vi "telemetry_beta.vi"() -> ()   [LabVIEW 2017]
uses:
  <vilib>/nican/nican.llb/ncNetAttr.ctl
  <vilib>/Platform/TimedLoop/XDataNode/XDataNode.xnode
  <vilib>/Platform/TimedLoop/XDataNode/nitl_modes.ctl
  <vilib>/Platform/TimedLoop/XDataNode/XDNodeRunTimeDep.lvlib
  <vilib>/Platform/TimedLoop/XDataNode/wakeup.ctl
  <vilib>/Platform/TimedLoop/XDataNode/timing_clust.ctl
panel:
  out "output cluster":T1
  in  "CAN1 Enable":bool
  in  "STOP":bool
  out "Error CAN1":errorcluster {"code" format="%.0x"}
  out "Error CAN0":errorcluster {"code" format="%.0x"}
  in  "Communication":u16(ring) items=["WiFi", "NI CAN", "NI XCAN"]
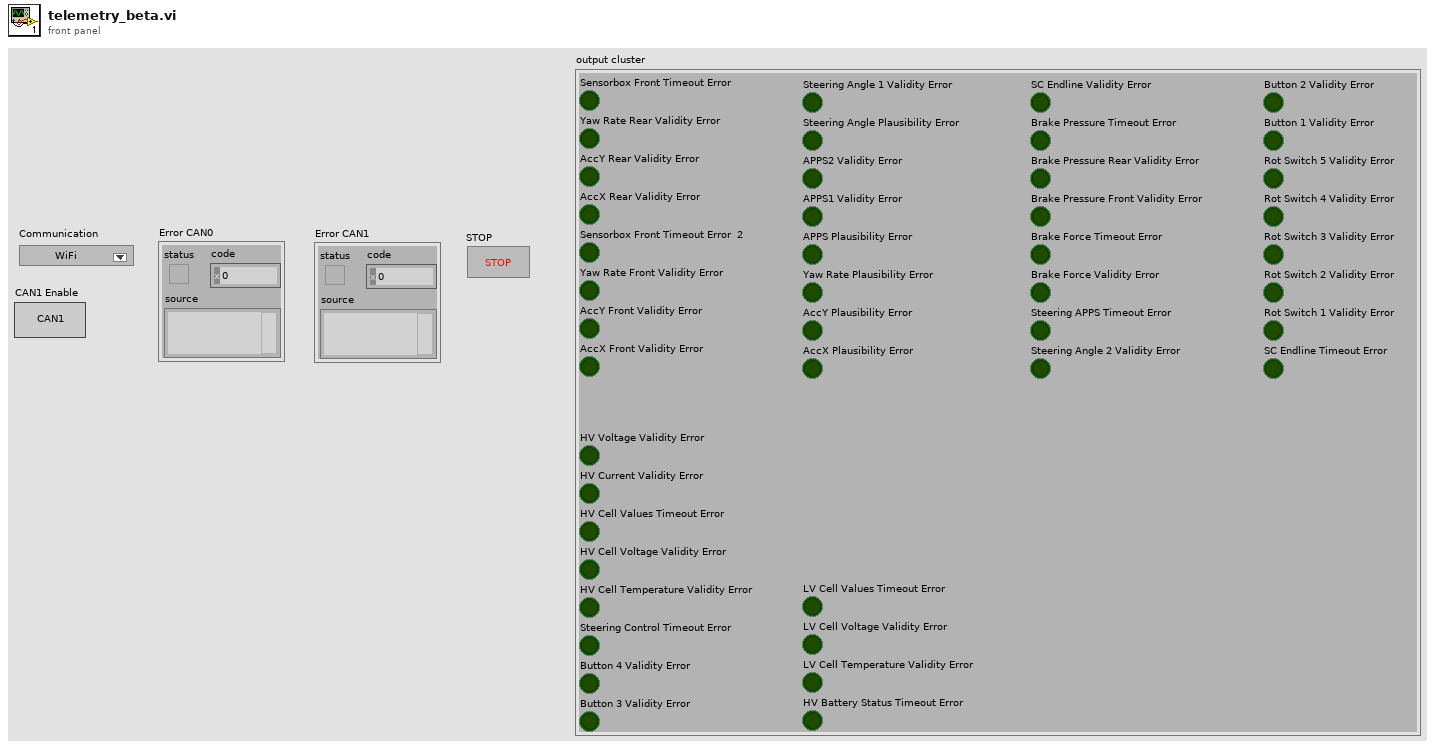
[diagram p1: front panel]
types:
  T1 = cluster{"Sensorbox Front Timeout Error ":bool, "Yaw Rate Rear Validity Error ":bool, "AccY Rear Validity Error":bool, "AccX Rear Validity Error ":bool, "Sensorbox Front Timeout Error  2":bool, "Yaw Rate Front Validity Error":bool, "AccY Front Validity Error":bool, "AccX Front Validity Error":bool, "Steering Angle 1 Validity Error":bool, "Steering Angle Plausibility Error":bool, "APPS2 Validity Error":bool, "APPS1 Validity Error":bool, "APPS Plausibility Error ":bool, "Yaw Rate Plausibility Error ":bool, "AccY Plausibility Error ":bool, "AccX Plausibility Error ":bool, "SC Endline Validity Error":bool, "Brake Pressure Timeout Error ":bool, "Brake Pressure Rear Validity Error":bool, "Brake Pressure Front Validity Error":bool, "Brake Force Timeout Error ":bool, "Brake Force Validity Error ":bool, "Steering APPS Timeout Error":bool, "Steering Angle 2 Validity Error":bool, "Button 2 Validity Error":bool, "Button 1 Validity Error":bool, "Rot Switch 5 Validity Error":bool, "Rot Switch 4 Validity Error":bool, "Rot Switch 3 Validity Error":bool, "Rot Switch 2 Validity Error":bool, "Rot Switch 1 Validity Error":bool, "SC Endline Timeout Error":bool, "HV Voltage Validity Error":bool, "HV Current Validity Error":bool, "HV Cell Values Timeout Error":bool, "HV Cell Voltage Validity Error":bool, "HV Cell Temperature Validity Error":bool, "Steering Control Timeout Error":bool, "Button 4 Validity Error":bool, "Button 3 Validity Error":bool, "LV Cell Values Timeout Error":bool, "LV Cell Voltage Validity Error":bool, "LV Cell Temperature Validity Error":bool, "HV Battery Status Timeout Error":bool}
  T2 = typedef "ncNetAttr.ctl" = cluster{"Start On Open":enum32{"FALSE", "TRUE"}, "Baud Rate":u32, "Read Queue Length":u32, "Write Queue Length":u32, "Standard Comparator":u32, "Standard Mask":u32, "Extended Comparator":u32, "Extended Mask":u32}
  T3 = typedef "xobjhandle.ctl" = u32
  T4 = cluster{"ObjHandle CAN0":T3, "Error CAN0":errorcluster, "Error CAN1":errorcluster, "ObjHandle CAN1":T3, "Double":bool}
  T5 = typedef "XDNodeRunTimeDep.lvlib/timing_clust.ctl" = cluster{"Expected End [f-1]":u64, "Actual End [f-1]":u64, "Finished Late? [f-1]":bool, "Expected End [i-1]":u64, "Actual End [i-1]":u64, "Finished Late? [i-1]":bool, "Expected Start [i]":u64, "Actual Start [i]":u64, "Expected Start [f]":u64, "Actual Start [f]":u64, "Source Name":string, "Structure Name":string, "Period":i64, "Deadline":i64, "Offset":i64, "Start":i64, "Priority":i32, "Timeout":i32, "Mode":T6, "Wakeup Reason":T7, "Error":errorcluster, "Source Type":string, "Secondary Source Type":string, "Global End Time":u64, "Global Start Time":u64, "Frame Duration":u64, "Iteration Duration":u64, "Assigned CPU":i32, "I/O Scan Engine Mode":u32}
  T6 = typedef "XDNodeRunTimeDep.lvlib/nitl_modes.ctl" = enum32{"No Change", "Process missed periods, maintain original phase", "Discard missed periods, maintain original phase", "Process missed periods, ignore original phase", "Discard missed periods, ignore original phase"}
  T7 = typedef "XDNodeRunTimeDep.lvlib/wakeup.ctl" = enum32{"Normal", "Aborted", "Asynchronous wakeup", "Timing source error", "Timed loop error", "Timeout"}
  T8 = typedef "CanFrameTimed.ctl" = cluster{"Timestamp":dbl, "ArbitrationId":u32, "IsRemote":u8, "DataLength":u8, "Data":u8[]}
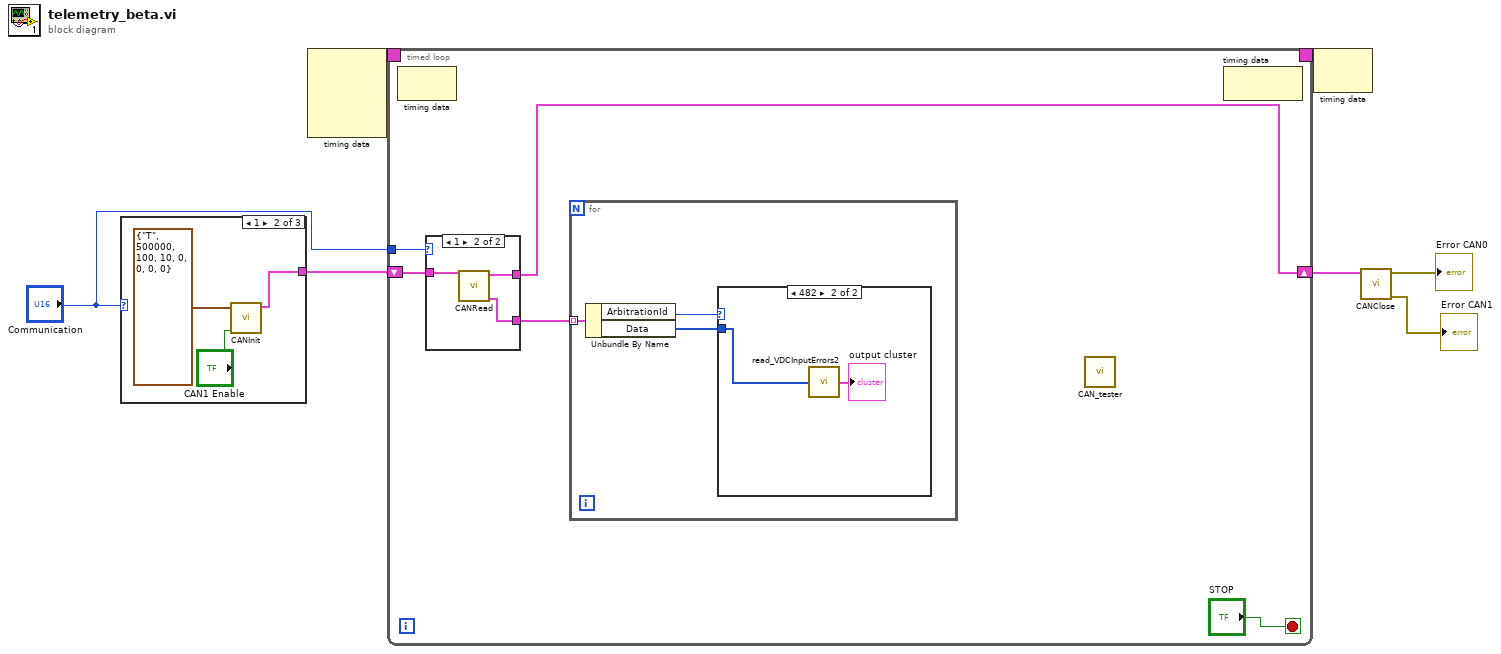
[diagram p0: block diagram]
diagram:
  n1 = case shown="1" "Communication" {
    tunnel: [_ w9 _] -> w5
    frame 0, Default {
    }
    frame 1 {
      n2 = call "CANInit.vi"("CAN1 Enable"="CAN1 Enable", "CAN Network Interface Config"=T2 {"Start On Open"=enum."TRUE", "Baud Rate"=500000, "Read Queue Length"=100, "Write Queue Length"=10, "Standard Comparator"=0, "Standard Mask"=0, "Extended Comparator"=0, "Extended Mask"=0}) -> ("Double CAN"=w9:T4)  [unwired: 9 in]
    }
    frame 2 {
    }
  }
  n3 = node-c288() -> (w7:T5)  [unwired: 4 in]
  n4 = timed-loop {
    timing: w7 -> [_]
    timing-out: [_] -> w6
    shift-right: [w14] -> w3
    shift-left: w5 -> [w15]
    tunnel: "Communication" -> [w13]
    stop <- "STOP" stop-if-true
    n5 = node-c288() -> ()  [unwired: 1 in, 1 out]
    n6 = case shown="1" w13 {
      tunnel: w15 -> [w21 w24]
      tunnel: [w21 w23] -> w14
      tunnel: [_ w22] -> w11
      frame 0, Default {
      }
      frame 1 {
        n7 = call "CANRead.vi"("Double CAN in"=w24) -> ("Data"=w22:T8[], "Double CAN out"=w23:T4)  [unwired: 9 in]
      }
    }
    n8 = for {
      tunnel: w11 -> [w18] mode=indexing
      n9 = Unbundle By Name(w18) -> ("ArbitrationId"=w17:u32, "Data"=w16:u8[])
      n10 = case shown="482" w17 {
        tunnel: w16 -> [_ w20]
        frame 0, Default {
        }
        frame 1154 {
          n11 = call "read_VDCInputErrors2.vi"("Array"=w20) -> ("output cluster"=→"output cluster":T1)
        }
      }
    }
    n12 = call "CAN_tester.vi"() -> ()  [unwired: 12 in]
    n13 = node-c288() -> ()  [unwired: 1 in, 1 out]
  }
  n14 = node-c288(w6) -> ()  [unwired: 1 out]
  n15 = call "CANClose.vi"("Double CAN in"=w3) -> ("Error CAN1"=→"Error CAN1":errorcluster, "Error CAN0"=→"Error CAN0":errorcluster)  [unwired: 9 in]
